vi "Remove Item Property.vi"(8 "error in (no error)":errorcluster, 10 "Property Name":string, 11 "Item Reference in":T1 format="%.0x") -> (0 "error out":errorcluster, 2 "removed":bool, 3 "Item Reference out":T1 format="%.0x")   [LabVIEW 2013, in "Hierarchy Framework.lvlib" / "Item.lvclass"]
doc: "Removes the property specified by <B>Property Name</B> from a custom device item."
uses:
  Item.lvclass
  Ctls/Item Reference.ctl
  Generic/Generic.lvclass
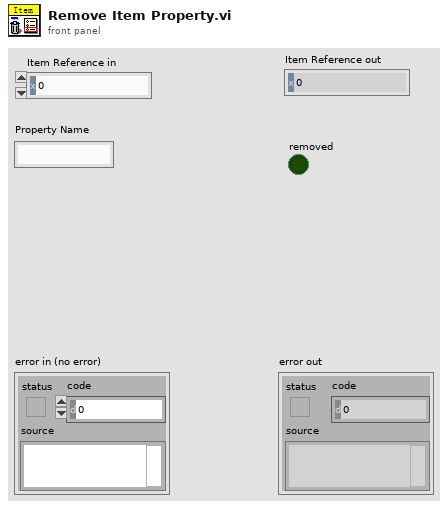
[diagram p1: front panel]
types:
  T1 = typedef "Hierarchy Framework.lvlib/Item.lvclass/Item Reference.ctl" = u64
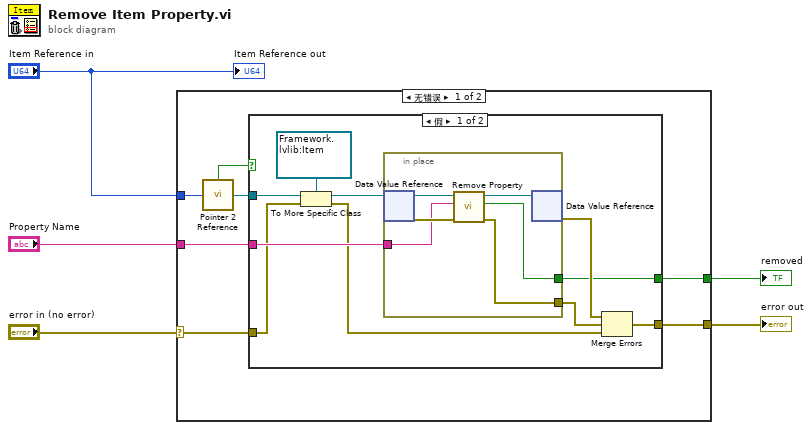
[diagram p0: block diagram]
diagram:
  n1 = case shown="无错误" "error in (no error)" {
    selector: "error in (no error)" -> [w10 w30]
    tunnel: "Item Reference in" -> [w8 _]
    tunnel: "Property Name" -> [w12 _]
    tunnel: [w11 w30] -> w3
    tunnel: [w9 _] -> w1
    frame No Error {
      n2 = call "Pointer 2 Reference.vi"("Pointer"=w8) -> ("Not A Refnum?"=w7:bool, "Generic Reference"=w6:refnum<data-value>)
      n3 = case shown="假" w7 {
        tunnel: w12 -> [w22 _]
        tunnel: w10 -> [w16 w29]
        tunnel: [w20 w29] -> w11
        tunnel: [w18 _] -> w9
        tunnel: w6 -> [w17 _]
        frame False {
          n4 = To More Specific Class(target class=refnum<data-value> refnum ("Item"), reference=w17, error in=w16) -> (specific class reference=w14:refnum<data-value>, error out=w13:errorcluster)
          n5 = in-place {
            in-place-border: w22 -> [w25]
            in-place-border: [w24] -> w19
            in-place-border: [w23] -> w18
            n6 = in-place-dvr #1(w14) -> (w28:refnum<class "Item.lvclass">, w26:errorcluster)
            n7 = call-dynamic "Remove Property.vi"("error in (no error)"=w26, "Property Name"=w25, "Item输入"=w28) -> ("error out"=w24:errorcluster, "removed"=w23:bool, "Item输出"=w27:refnum<class "Item.lvclass">)  [unwired: 6 in]
            n8 = in-place-dvr #1(w27) -> (w21:errorcluster)  [unwired: 1 out]
          }
          n9 = Merge Errors(w21, w19, w13) -> (w20:errorcluster)
        }
        frame True {
        }
      }
    }
    frame Error {
    }
  }
  "error out" <- w3
  "removed" <- w1
  "Item Reference out" <- "Item Reference in"
